vi "SVL Exp Avg Level (resampled) (1 Ch).vi"(6 "restart averaging (F)":bool, 8 "error in (no error)":errorcluster, 9 "exponential weighting":dbl=1.0 format="%.2f", 10 "even-angle channel info":T1={"channel name"="", "description"="", " channel info"={"sensor sensitivity"=1000.0, "engineering units"=1, "dB reference"=1.0, "custom label"="EU", "weighting filter"=0, "pregain"=0.0}} {"channel info"."pregain" format="%.2f"; "channel info"."weighting filter" items=["Linear", "A-weighting", "B-weighting", "C-weighting", "ITU-R 468-4", "Dolby", "CCITT", "C-message", "Wb", "Wc", "Wd", "We", "Wf", "Wh", "Wj", "Wk", "Wm", "AES17 20 kHz lowpass", "AES17 40 kHz lowpass", "AES17 20 kHz highpass", "AES17 40 kHz highpass"]; "channel info"."dB reference" format="%^.1e"; "channel info"."engineering units" items=["custom..."=0, "V"=1, "A"=21, "C"=30, "pC"=31, "s"=32, "-"=29, "Pa"=2, "N"=20, "g"=3, "m/s^2"=4, "m/s"=5, "m"=6, "mm/s"=12, "mm"=13, "micron/s"=14, "micron"=15, "in/s^2"=7, "in/s"=8, "in"=9, "mil/s"=10, "mil"=11, "rad/s^2"=16, "rad/s"=17, "rad"=18, "deg/s^2"=26, "deg/s"=27, "deg"=28, "RPM"=22, "cycle/s^2"=23, "Hz"=24, "cycle"=25, "strain"=19]; "channel info"."sensor sensitivity" format="%#_5f"}, 11 "even-angle signal [EU]":T5 {"even-angle signal" format="%.2f"; "dr" format="%.2f"; "r0" format="%.2f"}) -> (0 "error out":errorcluster, 2 "unit label":string, 3 "exp avg level [EU rms]":cluster{"r0":dbl, "dr":dbl, "level":dbl[]} {"level" format="%.2f"; "dr" format="%.2f"; "r0" format="%.2f"})   [LabVIEW 2017, in "SoundVib_VibrationLevel.lvlib"]
doc: "Computes the exponential averaged level of <B>scaled signal [EU]</B> or <B>even-angle signal [EU]</B>. <B>scaled signal [EU]</B> should have a zero DC component. You can attenuate the DC component with hardware AC-coupling filters and with software high-pass filters. Wire data to the <B>scaled signal [EU]</B> input to determine the polymorphic instance to use or manually select the instance."
uses:
  <vilib>/addons/Sound and Vibration/svt_Level/SoundVib_VibrationLevel.lvlib
  <vilib>/addons/_NISVFA/_Shared subVIs/Controls/svc_Resampled Channel Info.ctl
  <vilib>/addons/_NISVFA/_Shared subVIs/Controls/svc_Channel Info.ctl
  <vilib>/addons/_NISVFA/_Shared subVIs/Controls/svc_Engineering Units Text Ring.ctl
  <vilib>/addons/_NISVFA/_Shared subVIs/Controls/svc_Weighting Filter Text Ring.ctl
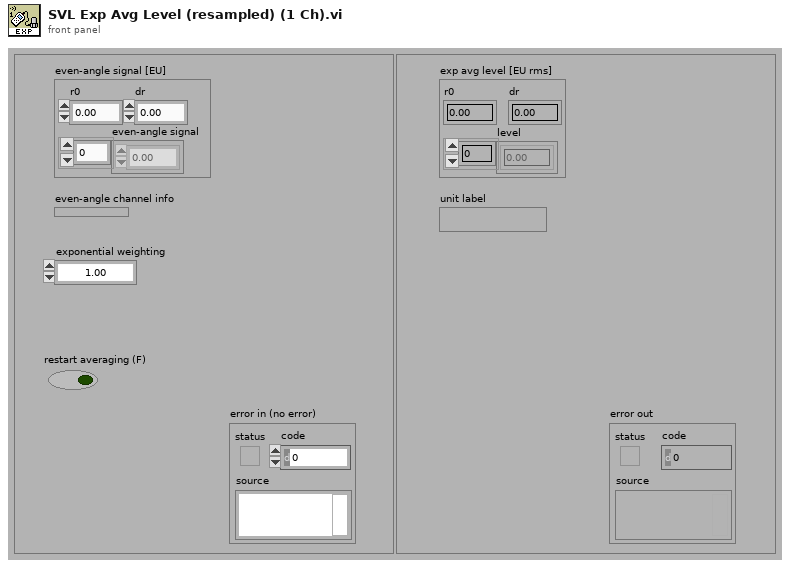
[diagram p1: front panel]
types:
  T1 = typedef "svc_Resampled Channel Info.ctl" = cluster{"channel name":string, "description":string, " channel info":T2}
  T2 = typedef "svc_Channel Info.ctl" = cluster{"sensor sensitivity":dbl, "engineering units":T3, "dB reference":dbl, "custom label":string, "weighting filter":T4, "pregain":dbl}
  T3 = typedef "svc_Engineering Units Text Ring.ctl" = u16
  T4 = typedef "svc_Weighting Filter Text Ring.ctl" = u16
  T5 = cluster{"r0":dbl, "dr":dbl, "even-angle signal":dbl[]}
  T6 = enum16{"RMS", "Running RMS", "Exp avg  ", "Dec exp avg ", "Peak", "Crest"}
  T7 = cluster{"r0":dbl, "dr":dbl, "even angle signal":dbl[]}
  T8 = enum16{"Reset filter", "Restart averaging", "Continue processing"}
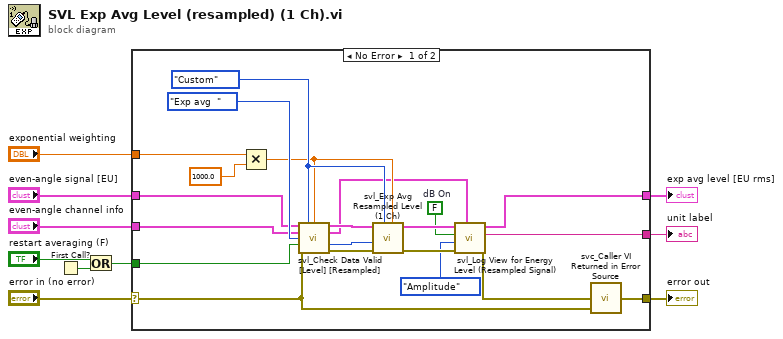
[diagram p0: block diagram]
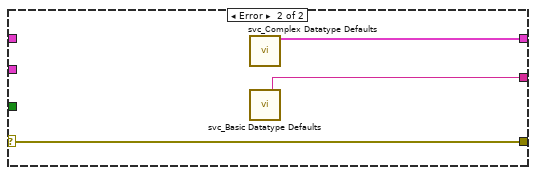
[diagram p2: hidden frame]
diagram:
  n1 = First Call?() -> (First Call?: T/F=w5:bool)
  n2 = Or(x="restart averaging (F)", y=w5) -> (x .or. y?=w4:bool)
  n3 = case shown="No Error" "error in (no error)" {
    selector: "error in (no error)" -> [w11 w34]
    tunnel: [w23 w34] -> w10
    tunnel: [w30 w33] -> w9
    tunnel: [w12 w32] -> w8
    tunnel: "even-angle signal [EU]" -> [w15 _]
    tunnel: w4 -> [w22 _]
    tunnel: "exponential weighting" -> [w19 _]
    tunnel: "even-angle channel info" -> [w14 _]
    frame No Error {
      w20 = enum16{"Slow", "Fast", "Impulse", "Custom"}."Custom" ("exponential mode")
      w27 = FALSE  # dB On
      n4 = Multiply(x=w19, y=1000.0) -> (x*y=w18:dbl)
      n5 = call <vilib>:"svl_Check Data Valid [Level] [Resampled].vi"("even angle signal"=w15, "exponential mode"=w20, "time constant [ms]"=w18, "even angle channel info"=w14, "Level Analysis"=T6."Exp avg  ", "restart averaging (F)"=w22, "error in (no error)"=w11) -> ("dup even angle signal"=w16:T7, "dup even angle channel info"=w13:T1, "processing state"=w24:T8, "error out"=w26:errorcluster)  [unwired: 5 in]
      n6 = call <vilib>:"svl_Exp Avg Resampled Level (1 Ch).vi"("timeConstant"=w18, "exponential mode"=w20, "error in (no error)"=w26, "processing state"=w24, "even angle signal"=w16) -> ("error out"=w29:errorcluster, "even angle signal"=w28:T7)  [unwired: 3 in, 2 out]
      n7 = call <vilib>:"svl_Log View for Energy Level (Resampled Signal).vi"("resampled channel info"=w13, "error in (no error)"=w29, "view mode"=enum16{"Power", "Amplitude"}."Amplitude", "dB On (T)"=w27, "even angle signal"=w28) -> ("error out"=w31:errorcluster, "unit label"=w30:string, "even angle signal"=w12:T7)  [unwired: 4 in]
      n8 = call <vilib>:"svc_Caller VI Returned in Error Source.vi"("warning input to caller"=w11, "error in (no error)"=w31) -> ("error out"=w23:errorcluster)  [unwired: 3 in]
    }
    frame Error {
      n9 = call <vilib>:"svc_Complex Datatype Defaults.vi"() -> ("empty spectrum"=w32:cluster{"f0":dbl, "df":dbl, "magnitude":dbl[]})  [unwired: 11 in, 8 out]
      n10 = call <vilib>:"svc_Basic Datatype Defaults.vi"() -> ("empty string"=w33:string)  [unwired: 7 in, 12 out]
    }
  }
  "exp avg level [EU rms]" <- w8
  "unit label" <- w9
  "error out" <- w10
